vi "controll.vi"   [LabVIEW 2016]
uses:
  <vilib>/NXT/Block Support/NXT_ButtonSelector.ctl
  <vilib>/NXT/Block Support/NXT_InputPort.ctl
  <vilib>/NXT/Block Support/NXT_OutputPort.ctl
  <vilib>/NXT/Dual Mode Library/Sensors/readNXTButton.vi
  <vilib>/NXT/Dual Mode Library/Waits/Wait_Num.vi
  <vilib>/NXT/NXTIO Xnodes/NXTIONodeSubVIs/NXTStopMotors.vi
  <vilib>/NXT/Dual Mode Library/Sensors/EV3_Infrared_Remote.vi
  <vilib>/NXT/NXTIO Xnodes/NXTIONodeSubVIs/NXTMoveMotors.vi
  <vilib>/NXT/NXTIO Xnodes/AddressXNode/NXTIOAddress.xnode
  <vilib>/NXT/NXTIO Xnodes/NXTIOXNode/NXTIO.xnode
  <vilib>/NXT/Subs/LVHSConnector.ctl
  <vilib>/NXT/LegoClasses/BrickReference/BrickReference.lvclass
types:
  T1 = typedef "NXT_OutputPort.ctl" = u8
  T2 = typedef "NXT_InputPort.ctl" = u32
  T3 = typedef "NXT_ButtonSelector.ctl" = u16
  T4 = typedef "LVHSConnector.ctl" = refnum<class "BrickReference.lvclass">
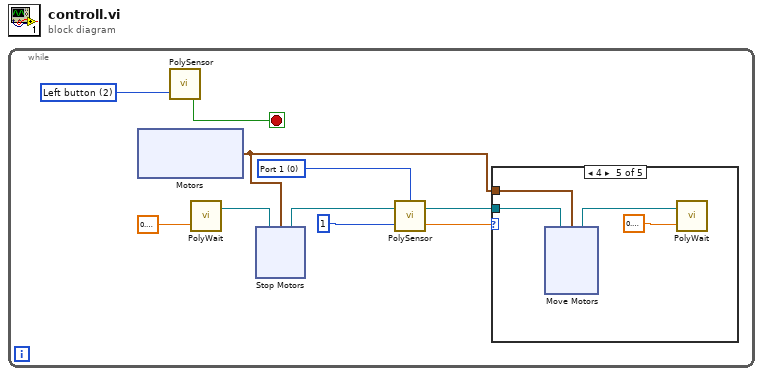
[diagram p0: block diagram]
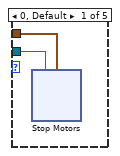
[diagram p2: hidden frame]
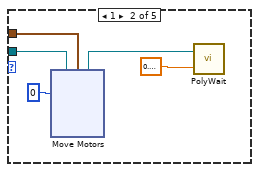
[diagram p3: hidden frame]
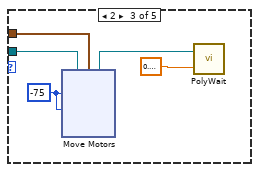
[diagram p4: hidden frame]
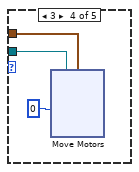
[diagram p5: hidden frame]
diagram:
  n1 = while {
    stop <- w10 stop-if-true
    w5 = T2 0 items=["Port 1", "Port 2", "Port 3", "Port 4"] ("Port (Port 1)")
    w9 = T3 2 items=["Enter button"=3, "Left button"=2, "Right button"=1, "Up Button"=4, "Down Button"=5] ("Button (Enter button)")
    n2 = xnode "Motors"() -> ("Motor"=w1:cluster{"Port":T1, "Port":T1})
    n3 = call-poly <vilib>:"PolySensor.vi"("Button (Enter button)"=w9) -> ("Yes/No"=w10:bool)  [unwired: 2 in, 1 out]
    n4 = call-poly <vilib>:"PolyWait.vi"("Time (1 sec)"=sgl 0.1) -> ("NXT/EV3"=w7:T4)  [unwired: 3 in]
    n5 = xnode "Stop Motors"("Motors"=w1, "NXT/EV3"=w7) -> ("NXT/EV3"=w6:T4)
    n6 = call-poly <vilib>:"PolySensor.vi"("Channel"=u8 1, "NXT/EV3"=w6, "Port (Port 1)"=w5) -> ("Button Detected"=w3:sgl, "NXT/EV3"=w2:T4)
    n7 = case shown="4" w3 {
      tunnel: w2 -> [w13 w23 w36 w46 w58]
      tunnel: w1 -> [w12 w19 w35 w47 w59]
      frame 0, Default {
        n8 = xnode "Stop Motors"("Motors"=w12, "NXT/EV3"=w13) -> ()  [unwired: 1 out]
      }
      frame 1 {
        n9 = xnode "Move Motors"("Power/Speed 1"=i8 0 ("Power/Speed 2"), "Motors"=w19, "NXT/EV3"=w23) -> ("NXT/EV3"=w22:T4)  [unwired: 1 in]
        n10 = call-poly <vilib>:"PolyWait.vi"("Time (1 sec)"=sgl 0.1, "NXT/EV3"=w22) -> ()  [unwired: 2 in, 1 out]
      }
      frame 2 {
        w34 = i8 -75 ("Power/Speed 1")
        n11 = xnode "Move Motors"("Power/Speed 2"=w34, "Power/Speed 1"=w34, "Motors"=w35, "NXT/EV3"=w36) -> ("NXT/EV3"=w33:T4)
        n12 = call-poly <vilib>:"PolyWait.vi"("Time (1 sec)"=sgl 0.1, "NXT/EV3"=w33) -> ()  [unwired: 2 in, 1 out]
      }
      frame 3 {
        n13 = xnode "Move Motors"("Power/Speed 2"=i8 0, "Motors"=w47, "NXT/EV3"=w46) -> ()  [unwired: 1 in, 1 out]
      }
      frame 4 {
        n14 = xnode "Move Motors"("Motors"=w59, "NXT/EV3"=w58) -> ("NXT/EV3"=w57:T4)  [unwired: 2 in]
        n15 = call-poly <vilib>:"PolyWait.vi"("Time (1 sec)"=sgl 0.1, "NXT/EV3"=w57) -> ()  [unwired: 2 in, 1 out]
      }
    }
  }
